vi "time4.vi"() -> ()   [LabVIEW 2020]
panel:
  out "time 4":T1
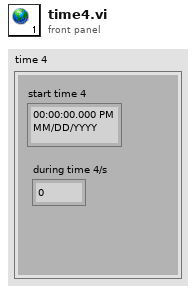
[diagram p1: front panel]
types:
  T1 = cluster{"start time 4":timestamp, "during time 4/s":dbl}
diagram:
